vi "Set_Thermistor_Offset.vi"() -> ()   [LabVIEW 2022 SP3]
uses:
  Sub VIs/ADAM Controls/Channel_names.ctl
  <vilib>/Analysis/NI_AALBase.lvlib
  <vilib>/Analysis/baseanly.llb/Mean (DBL).vi
  Sub VIs/ADAM Controls/Calib_type_ADAM.ctl
  Sub VIs/ADAM Controls/Module_type_ADAM.ctl
panel:
  out "After Tweak":dbl[][](graph)
  in  "Apply Offset":bool
  in  "Stop Looping":bool
  out "Current Offset\n\nTweak required":dbl[][](array[numeric]) format="%#.5f"
  out "Current Offset":dbl[][](graph)
  in  "History Length (mins)":dbl=2.0
  out "Selected Channel Names":string[](array[string])
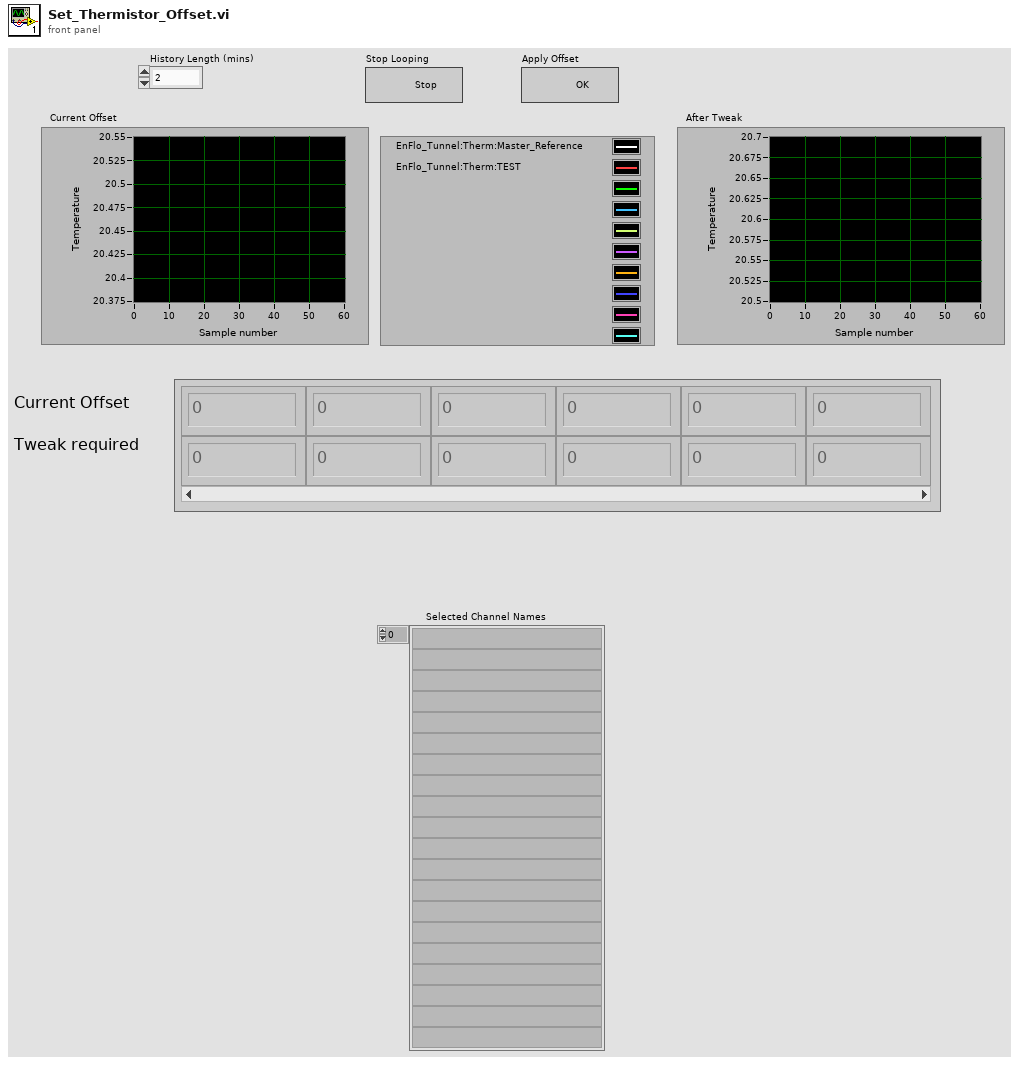
[diagram p1: front panel]
types:
  T1 = enum16{"Zero or one", "One", "Zero or more", "One or more"}
  T2 = typedef "Channel_names.ctl" = enum16{"Active Only", "Active + Off", "All Channels", "Changeable Only"}
  T3 = typedef "Module_type_ADAM.ctl" = string
  T4 = typedef "Ch_description_ADAM.ctl" = cluster{"Ch Name":string, "Type":T3, "Function":T5, "Ch State":T6, "Calibration type":T7, "A":dbl, "B":dbl, "C":dbl, "D":dbl, "Comments":string, "Address":T8, "String":string, "Duty":u16}
  T5 = typedef "Function_ADAM.ctl" = enum16{"Analogue Input", "Digital Input", "Event counter", "Event rate", "Analogue Output", "Digital Output", "Relay Output"}
  T6 = typedef "Channel_State.ctl" = enum16{"On", "Off", "Always On", "Always Off"}
  T7 = typedef "Calib_type_ADAM.ctl" = string
  T8 = typedef "Address.ctl" = cluster{"Main":i32, "Ch.":i32, "Sub":i32, "Port Name":string}
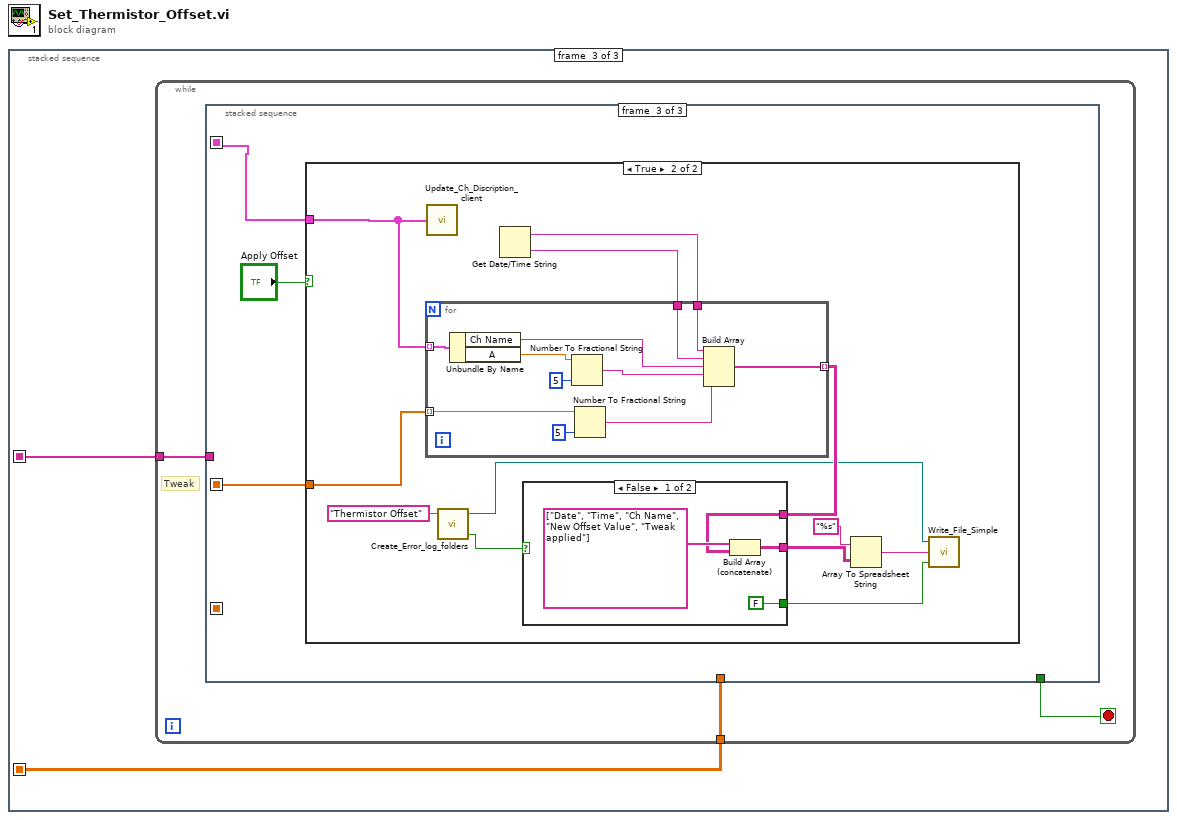
[diagram p0: block diagram]
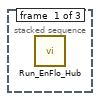
[diagram p2: hidden frame]
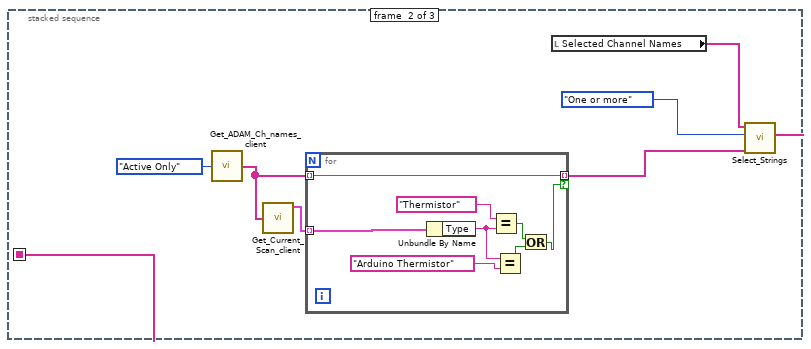
[diagram p3: hidden frame]
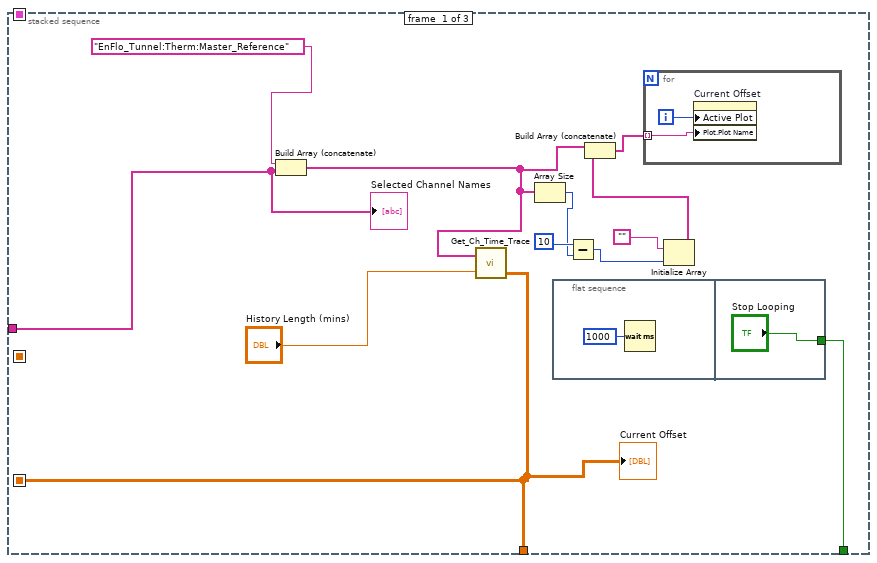
[diagram p4: hidden frame]
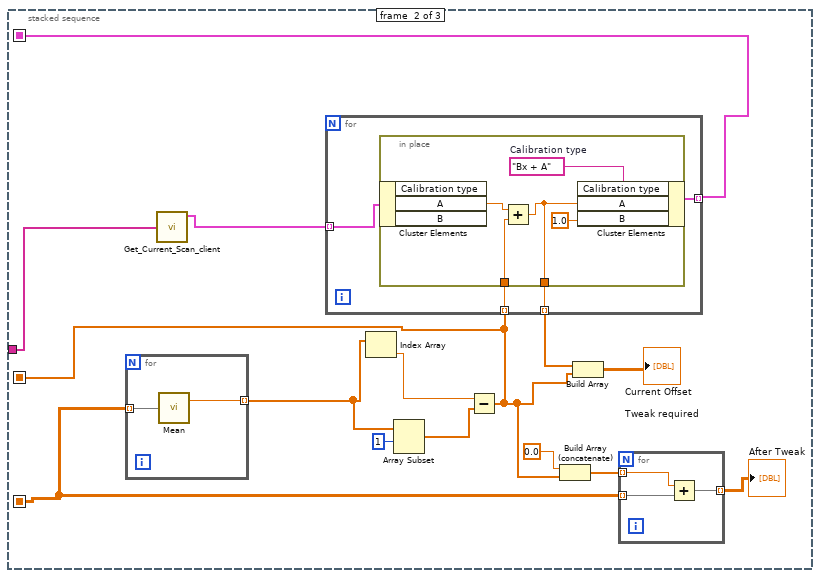
[diagram p5: hidden frame]
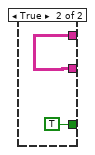
[diagram p7: hidden frame]
diagram:
  n1 = stacked-sequence {
    seq-local: [_ _ w17] -> [_ _ _]
    seq-local: [_ w1 _] -> [_ _ w16]
    frame #0 {
      n2 = call "Run_EnFlo_Hub.vi"() -> ()  [unwired: 7 in, 1 out]
    }
    frame #1 {
      n3 = call "Get_ADAM_Ch_names_client.vi"("Channel names set"=Channel_names."Active Only") -> ("Ch names"=w2:string[])
      n4 = call "Get_Current_Scan_client.vi"("ADAM Ch Names"=w2) -> ("Ch Description Array"=w4:T4[])  [unwired: 1 in, 2 out]
      n5 = for {
        tunnel: w4 -> [w15] mode=indexing
        tunnel: [w9] -> w3 mode=indexing if=w8
        tunnel: w2 -> [w9] mode=indexing
        n6 = Unbundle By Name(w15) -> ("Type"=w13:T3)
        n7 = Equal?(x=T3 "Thermistor" ("Type"), y=w13) -> (x = y?=w11:bool)
        n8 = Equal?(x=w13, y=T3 "Arduino Thermistor" ("Type")) -> (x = y?=w10:bool)
        n9 = Or(x=w11, y=w10) -> (x .or. y?=w8:bool)
      }
      n10 = local read "Selected Channel Names"() -> (w5:string[])
      n11 = call "Select_Strings.vi"("Available Ch names"=w3, "Selector mode"=T1."One or more", "Desired Ch names (in)"=w5) -> ("Selected Channel Names"=w1:string[])  [unwired: 3 in, 2 out]
    }
    frame #2 {
      n12 = while {
        tunnel: [w20] -> w17
        tunnel: w16 -> [w19]
        stop <- w18 stop-if-true
        # "Tweak"
        n13 = stacked-sequence {
          seq-local: [w28 _ _] -> [_ w42 _]
          seq-local: [_ w38 _] -> [_ _ w66]
          seq-local: [_ w37 _] -> [_ _ w65]
          tunnel: [w28 _ _] -> w20
          tunnel: w19 -> [w30 w45 _]
          tunnel: [w29 _ _] -> w18
          frame #0 {
            n14 = Build Array (concatenate)("EnFlo_Tunnel:Therm:Master_Reference", w30) -> (w24:string[])
            n15 = call "Get_Ch_Time_Trace.vi"("Desired Ch Names"=w24, "History Length (mins)"="History Length (mins)") -> ("Output array"=w28:dbl[][])  [unwired: 2 out]
            "Current Offset" <- w28
            n16 = Array Size(array=w24) -> (size(s)=w22:i32)
            n17 = flat-sequence {
              tunnel: ["Stop Looping"] -> w29
              frame #0 {
                n18 = Wait (ms)(milliseconds to wait=u32 1000) -> ()  [unwired: 1 out]
              }
              frame #1 {
              }
            }
            n19 = Subtract(x=10 ("dimension size"), y=w22) -> (x-y=w21:i32)
            n20 = Initialize Array("", w21) -> (w25:string[])
            n21 = Build Array (concatenate)(w24, w25) -> (w26:string[])
            n22 = for {
              tunnel: w26 -> [w35] mode=indexing
              i -> [w36]
              n23 = property on="Current Offset" class="WFGraph (strict)"("Active Plot"=w36, "Plot.Plot Name"=w35) -> ()  [unwired: 2 in, 2 out]
            }
            "Selected Channel Names" <- w30
          }
          frame #1 {
            n24 = for {
              tunnel: w42 -> [w55] mode=indexing
              tunnel: [w54] -> w46 mode=indexing
              n25 = call-poly <vilib>:"Mean.vi"("X"=w55) -> ("mean"=w54:dbl)  [unwired: 1 out]
            }
            n26 = call "Get_Current_Scan_client.vi"("ADAM Ch Names"=w45) -> ("Ch Description Array"=w47:T4[])  [unwired: 1 in, 2 out]
            n27 = Index Array(array=w46) -> (element=w49:dbl)  [unwired: 1 in]
            n28 = Array Subset(array=w46, index=1) -> (w48:dbl[])  [unwired: 1 in]
            n29 = Subtract(x=w49, y=w48) -> (x-y=w37:dbl[])
            n30 = for {
              tunnel: w47 -> [w59] mode=indexing
              tunnel: w37 -> [w58] mode=indexing
              tunnel: [w57] -> w38 mode=indexing
              tunnel: [w56] -> w40 mode=indexing
              n31 = in-place {
                in-place-border: w58 -> [w63]
                in-place-border: [w61] -> w56
                w60 = T7 "Bx + A"  # Calibration type
                n32 = in-place-cluster #1(w59) -> ("A"=w64:dbl)  [unwired: 2 out]
                n33 = Add(x=w64, y=w63) -> (x+y=w61:dbl)
                n34 = in-place-cluster #1("Calibration type"=w60, "A"=w61, "B"=1.0) -> (w57:T4)
              }
            }
            n35 = Build Array (concatenate)(0.0, w37) -> (w43:dbl[])
            n36 = Build Array(w40, w37) -> (→"Current Offset\n\nTweak required":dbl[][])
            n37 = for {
              tunnel: w43 -> [w53] mode=indexing
              tunnel: w42 -> [w52] mode=indexing
              tunnel: [w51] -> w41 mode=indexing
              n38 = Add(x=w53, y=w52) -> (x+y=w51:dbl[])
            }
            "After Tweak" <- w41
          }
          frame #2 {
            n39 = case shown="True" "Apply Offset" {
              tunnel: w66 -> [_ w79]
              tunnel: w65 -> [_ w78]
              frame False {
              }
              frame True {
                n40 = call "Update_Ch_Discription_client.vi"("Channels to update In"=w79) -> ()  [unwired: 1 in]
                n41 = call "Create_Error_log_folders.vi"("Log Filename"="Thermistor Offset") -> ("Local Log File"=w68:path, "exists?"=w74:bool)  [unwired: 5 in]
                n42 = Get Date/Time String() -> (date string=w77:string, time string=w76:string)  [unwired: 3 in]
                n43 = for {
                  tunnel: w79 -> [w96] mode=indexing
                  tunnel: w78 -> [w92] mode=indexing
                  tunnel: w77 -> [w91]
                  tunnel: w76 -> [w90]
                  tunnel: [w86] -> w73 mode=indexing
                  n44 = Unbundle By Name(w96) -> ("Ch Name"=w89:string, "A"=w95:dbl)
                  n45 = Number To Fractional String(number=w95, precision (6)=i16 5) -> (F-format string=w88:string)  [unwired: 2 in]
                  n46 = Number To Fractional String(number=w92, precision (6)=i16 5) -> (F-format string=w87:string)  [unwired: 2 in]
                  n47 = Build Array(w91, w90, w89, w88, w87) -> (w86:string[])
                }
                n48 = case shown="False" w74 {
                  tunnel: w73 -> [w82 w85]
                  tunnel: [w81 w85] -> w72
                  tunnel: [FALSE ("append to file? (new file:F)") TRUE ("append to file? (new file:F)")] -> w70
                  frame False {
                    n49 = Build Array (concatenate)(string[] ["Date", "Time", "Ch Name", "New Offset Value", "Tweak applied"], w82) -> (w81:string[][])
                  }
                  frame True {
                  }
                }
                n50 = Array To Spreadsheet String(array=w72, 3:"%s" ("format string")) -> (spreadsheet string=w69:string)  [unwired: 1 in]
                n51 = call "Write_File_Simple.vi"("append to file? (new file:F)"=w70, "character string"=w69, "file path"=w68) -> ()  [unwired: 2 out]
              }
            }
          }
        }
      }
    }
  }
